vi "OnValueChange_leftUserTwo.vi"(8 "error in (no error)":errorcluster, 9 "Value":bool, 10 "Engine":refnum<class "Engine.lvclass">, 11 "Game in":refnum<class "Game.lvclass">) -> (0 "error out":errorcluster, 2 "Engine out":refnum<class "Engine.lvclass">, 3 "Game out":refnum<class "Game.lvclass">)   [LabVIEW 2019, in "RT_Game.lvlib" / "Game.lvclass"]
uses:
  Game.lvclass
  Engine/Engine.lvclass
  Engine/ChangeVolumeData.ctl
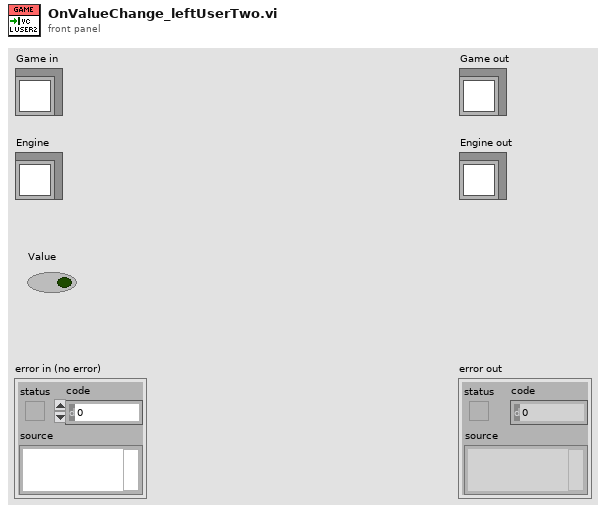
[diagram p1: front panel]
types:
  T1 = typedef "RT_Game.lvlib/Engine.lvclass/ChangeVolumeData.ctl" = enum16{"up", "down", "mute"}
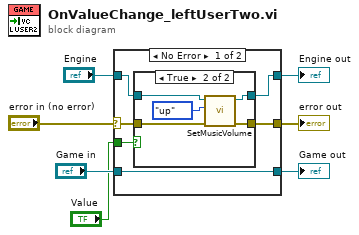
[diagram p0: block diagram]
diagram:
  n1 = case shown="No Error" "error in (no error)" {
    selector: "error in (no error)" -> [w12 w23]
    tunnel: [w11 w23] -> w6
    tunnel: [w13 w22] -> w4
    tunnel: "Game in" -> [w13 w22]
    tunnel: "Engine" -> [w10 w21]
    tunnel: [w9 w21] -> w2
    tunnel: "Value" -> [w8 _]
    frame No Error {
      n2 = case shown="True" w8 {
        tunnel: w12 -> [w14 w20]
        tunnel: [w14 w19] -> w11
        tunnel: w10 -> [w15 w18]
        tunnel: [w15 w17] -> w9
        frame False {
        }
        frame True {
          n3 = call "SetMusicVolume.vi"("error in (no error)"=w20, "VolumeData"=ChangeVolumeData."up", "Engine in"=w18) -> ("error out"=w19:errorcluster, "Engine out"=w17:refnum<class "Engine.lvclass">)  [unwired: 7 in]
        }
      }
    }
    frame Error {
    }
  }
  "error out" <- w6
  "Game out" <- w4
  "Engine out" <- w2
